vi "Speed PI Control.vi"() -> ()   [LabVIEW 2016]
panel:
  in  "I-Gain":dbl(slide)=1.0 scale=0.0..2.0
  in  "P-Gain":dbl(slide)=1.0 scale=0.0..2.0
  in  "Setpoint Speed (rps)":dbl(slide) scale=-8.3..8.3
  out "Speed (rps)":dynamicdata(graph)
  in  "stop (F)":bool
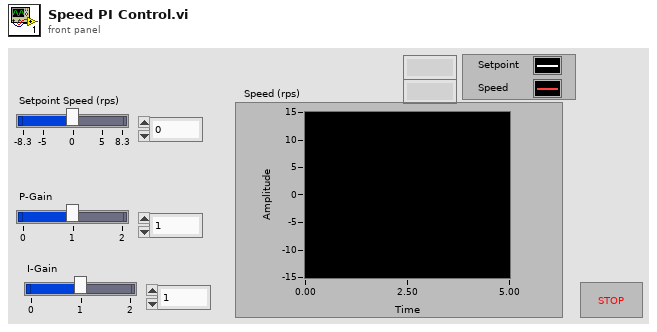
[diagram p1: front panel]
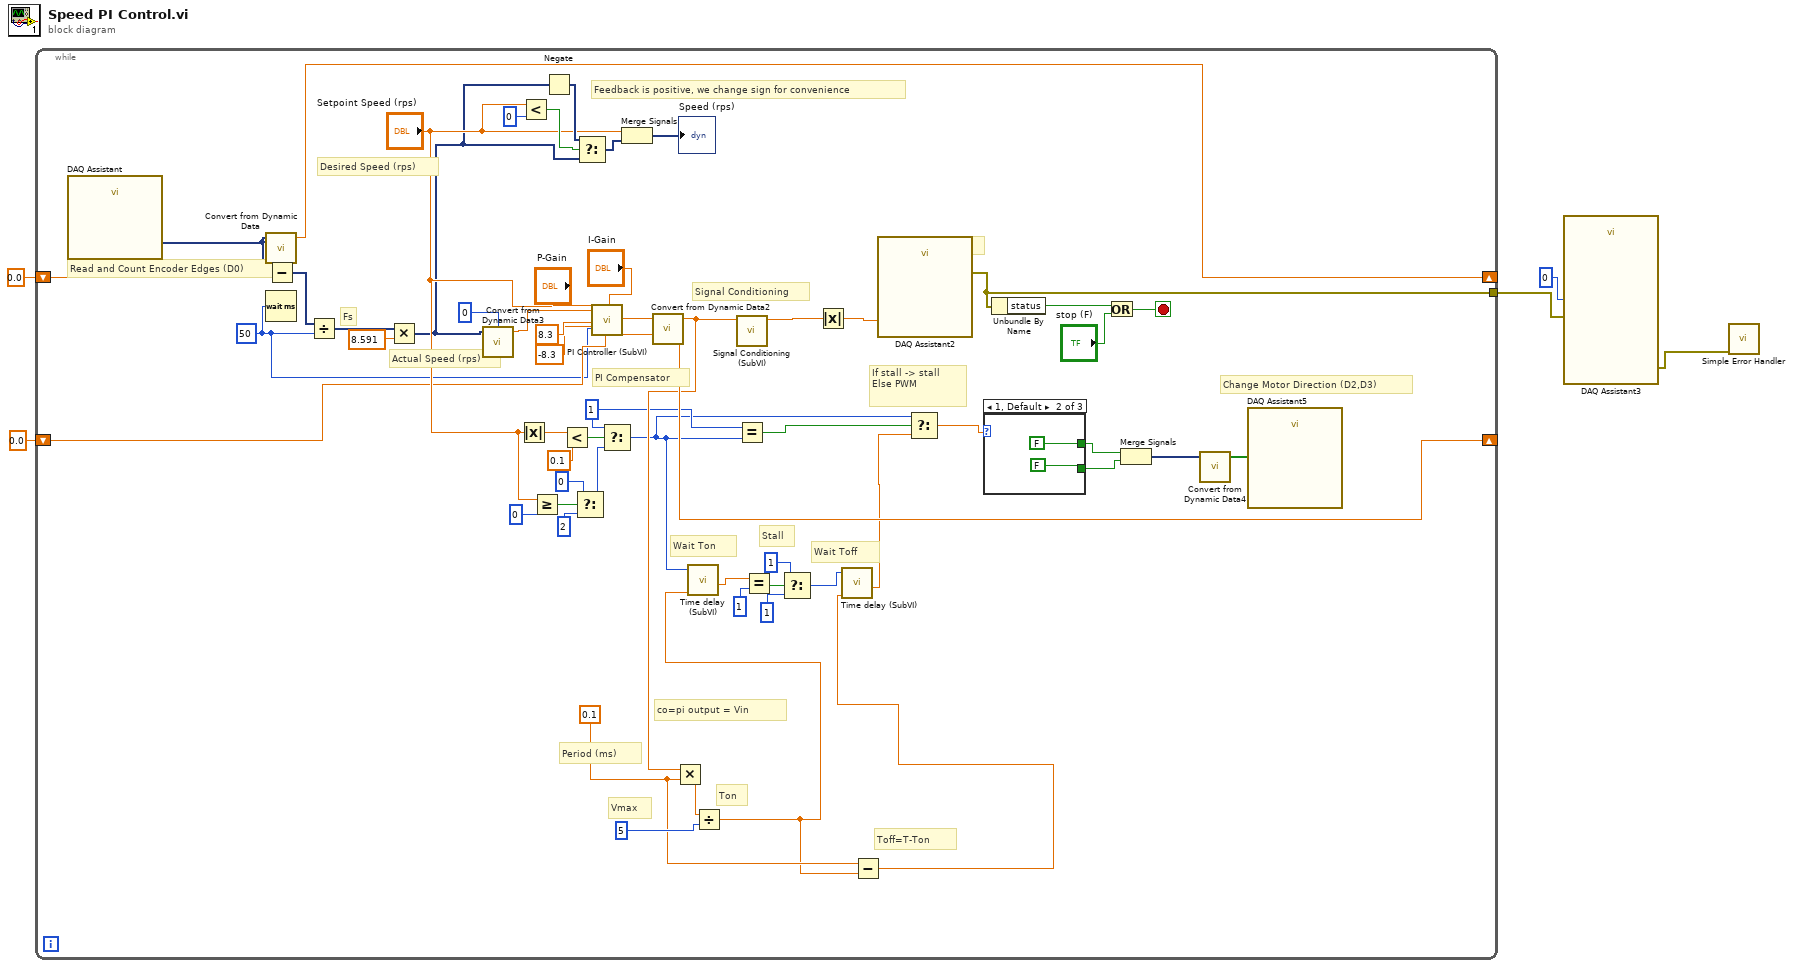
[diagram p0: block diagram]
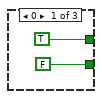
[diagram p2: hidden frame]
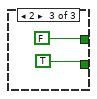
[diagram p3: hidden frame]
diagram:
  n1 = while {
    shift-right: [w63] -> _
    shift-left: 0.0 -> [w62]
    tunnel: [w58] -> w4
    shift-right: [w26] -> _
    shift-left: 0.0 -> [w29]
    stop <- w57 stop-if-true
    w22 = 0.1
    w18 = 1
    w28 = 50
    # "If stall -> stall\nElse PWM"
    # "Wait Toff"
    # "Stall"
    # "Wait Ton"
    # "Toff=T-Ton"
    # "Ton"
    # "Vmax"
    # "co=pi output = Vin"
    # "Period (ms)"
    # "Desired Speed (rps)"
    # "Feedback is positive, we change sign for convenience"
    # "Change Motor Direction (D2,D3)"
    # "Signal Conditioning"
    # "PI Compensator"
    # "Fs"
    # "Actual Speed (rps)"
    # "Read and Count Encoder Edges (D0)"
    # "Plant Input (Ao0)"
    n2 = call "DAQ Assistant"() -> ("data"=w54:dynamicdata)  [unwired: 16 in, 3 out]
    n3 = call "Convert from Dynamic Data"("Dynamic Data Type"=w54) -> ("Scalar"=w63:dbl)  [unwired: 3 in]
    n4 = Wait (ms)(milliseconds to wait=w28) -> ()  [unwired: 1 out]
    n5 = Subtract(x=w54, y=w62) -> (x-y=w61:dynamicdata)
    n6 = Divide(x=w61, y=w28) -> (x/y=w60:dynamicdata)
    n7 = Multiply(x=w60, y=8.591) -> (x*y=w27:dynamicdata)
    n8 = call "Convert from Dynamic Data3"("Dynamic Data Type"=w27, "Channel"=0) -> ("Scalar"=w34:dbl)  [unwired: 2 in]
    n9 = Absolute Value(x="Setpoint Speed (rps)") -> (abs(x)=w46:dbl)
    n10 = Less?(x="Setpoint Speed (rps)", y=0) -> (x < y?=w37:bool)
    n11 = Greater Or Equal?(x="Setpoint Speed (rps)", y=0) -> (x >= y?=w49:bool)
    n12 = Negate(x=w27) -> (-x=w36:dynamicdata)
    n13 = Less?(x=w46, y=0.1) -> (x < y?=w44:bool)
    n14 = Select(t=0, s=w49, f=2) -> (s? t:f=w43:i32)
    n15 = Select(t=w36, s=w37, f=w27) -> (s? t:f=w38:dynamicdata)
    n16 = call "PI Controller (SubVI).vi"("sp"="Setpoint Speed (rps)", "pv"=w34, "maxim"=8.3, "minim"=-8.3, "p"="P-Gain", "errsum"=w29, "i"="I-Gain", "h"=w28) -> ("output variable"=w25:dbl, "errsum"=w26:dbl)  [unwired: 18 in]
    n17 = Select(t=w18, s=w44, f=w43) -> (s? t:f=w14:i32)
    n18 = Merge Signals("Setpoint Speed (rps)", w38) -> (→"Speed (rps)":dynamicdata)
    n19 = call "Convert from Dynamic Data2"("Dynamic Data Type"=w25) -> ("Scalar"=w21:dbl)  [unwired: 3 in]
    n20 = Multiply(x=w21, y=w22) -> (x*y=w24:dbl)
    n21 = Divide(x=w24, y=5) -> (x/y=w16:dbl)
    n22 = call "Time delay (SubVI).vi"("Delay Time"=w16, "input"=w14) -> ("Output"=w15:dbl)  [unwired: 7 in]
    n23 = call "Signal Conditioning (SubVI).vi"("Input"=w21) -> ("Output"=w41:dbl)  [unwired: 10 in]
    n24 = Equal?(x=w18, y=w14) -> (x = y?=w17:bool)
    n25 = Equal?(x=w15, y=1) -> (x = y?=w11:bool)
    n26 = Select(t=1, s=w11, f=1) -> (s? t:f=w8:i32)
    n27 = Absolute Value(x=w41) -> (abs(x)=w42:dbl)
    n28 = Subtract(x=w22, y=w16) -> (x-y=w9:dbl)
    n29 = call "Time delay (SubVI).vi"("Delay Time"=w9, "input"=w8) -> ("Output"=w7:dbl)  [unwired: 7 in]
    n30 = call "DAQ Assistant2"("data"=w42) -> ("error out"=w58:errorcluster)  [unwired: 17 in, 1 out]
    n31 = Select(t=w14, s=w17, f=w7) -> (s? t:f=w6:dbl)
    n32 = case shown="1, Default" w6 {
      tunnel: [TRUE FALSE FALSE] -> w20
      tunnel: [FALSE FALSE TRUE] -> w19
      frame 0 {
      }
      frame 1, Default {
      }
      frame 2 {
      }
    }
    n33 = Unbundle By Name(w58) -> ("status"=w55:bool)
    n34 = Or(x=w55, y="stop (F)") -> (x .or. y?=w57:bool)
    n35 = Merge Signals(w20, w19) -> (w52:dynamicdata)
    n36 = call "Convert from Dynamic Data4"("Dynamic Data Type"=w52) -> ("Array"=w51:bool[])  [unwired: 3 in]
    n37 = call "DAQ Assistant5"("data"=w51) -> ()  [unwired: 17 in, 2 out]
  }
  n38 = call "DAQ Assistant3"("data"=0, "error in"=w4) -> ("error out"=w2:errorcluster)  [unwired: 16 in, 1 out]
  n39 = call <vilib>:"Simple Error Handler.vi"("error in (no error)"=w2) -> ()  [unwired: 4 in, 5 out]
